vi "add_automatic_steps.vi"(7 "references":T1, 8 "error in (no error)":errorcluster, 11 "automatic_steps":variant) -> (0 "error out":errorcluster)   [LabVIEW 2015, in "repub-dvr_nre.lvlib"]
uses:
  repub-dvr_nre.lvlib
  _controls/references.ctl
  private/_controls/input.ctl
  private/_controls/input_command.ctl
  private/_controls/output.ctl
  private/_controls/data.ctl
  _controls/configuration.ctl
  lv-recipe-machine/private/_controls/recipe_data.ctl
  lv-recipe-machine/public/_controls/mode.ctl
  lv-recipe-machine/public/_controls/manual_state.ctl
  lv-recipe-machine/public/_controls/automatic_state.ctl
  <userlib>/antonio-alexander/lv-waitgroup/public/_controls/api_waitgroup.ctl
  _controls/change.ctl
  lv-recipe-machine/lv-recipe-machine.lvlib
  <userlib>/antonio-alexander/lv-waitgroup/lv-waitgroup.lvlib
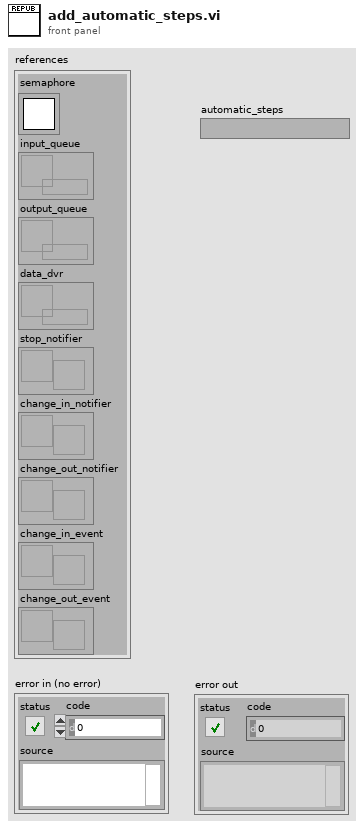
[diagram p1: front panel]
types:
  T1 = typedef "repub-dvr_nre.lvlib/references.ctl" = cluster{"semaphore":T2, "input_queue":refnum<queue>, "output_queue":refnum<queue>, "data_dvr":refnum<data-value>, "stop_notifier":refnum<notifier>, "change_in_notifier":refnum<notifier>, "change_out_notifier":refnum<notifier>, "change_in_event":refnum<user-event>, "change_out_event":refnum<user-event>}
  T2 = typedef "Semaphore RefNum" = refnum<k1>
  T3 = typedef "repub-dvr_nre.lvlib/data.ctl" = cluster{"configuration":T4, "working":cluster{"initialized":bool, "recipe_data":T5, "api_waitgroup":T9}}
  T4 = typedef "repub-dvr_nre.lvlib/configuration.ctl" = cluster{dbl}
  T5 = typedef "lv-recipe-machine.lvlib/recipe_data.ctl" = cluster{"mode":T6, "manual_state":T7, "automatic_state":T8, "step":string, "automatic_recipe":variant, "manual_actions":variant}
  T6 = typedef "lv-recipe-machine.lvlib/mode.ctl" = enum16{"<mode>", "manual", "automatic", "<null>"}
  T7 = typedef "lv-recipe-machine.lvlib/manual_state.ctl" = enum16{"<manual_state>", "failed", "action", "running", "idle", "<null>"}
  T8 = typedef "lv-recipe-machine.lvlib/automatic_state.ctl" = enum16{"<automatic_state>", "failed", "idle", "running", "paused", "transition", "stopped", "<null>"}
  T9 = typedef "lv-waitgroup.lvlib/api_waitgroup.ctl" = cluster{"waitgroups":refnum<data-value>, "waitgroup":string}
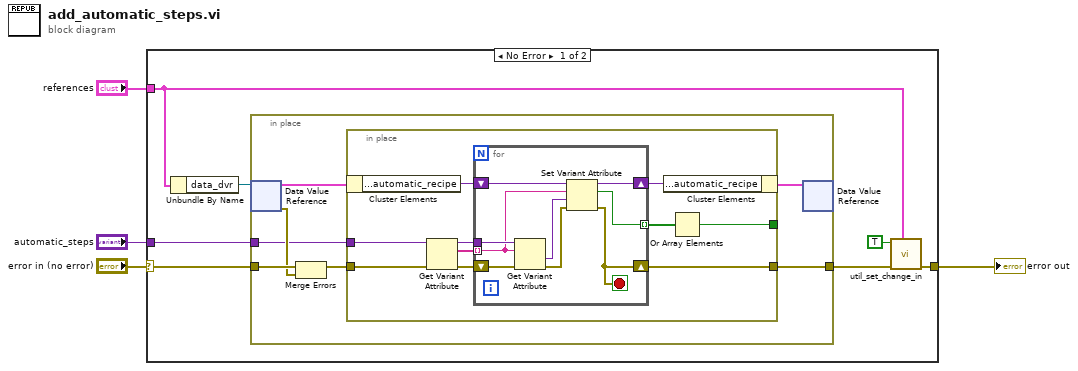
[diagram p0: block diagram]
diagram:
  n1 = case shown="No Error" "error in (no error)" {
    selector: "error in (no error)" -> [w10 w38]
    tunnel: [w8 w38] -> w1
    tunnel: "references" -> [w9 _]
    tunnel: "automatic_steps" -> [w7 _]
    frame No Error {
      n2 = Unbundle By Name(w9) -> ("data_dvr"=w11:refnum<data-value>)
      n3 = in-place {
        in-place-border: [w12] -> w6
        in-place-border: w10 -> [w18]
        in-place-border: w7 -> [w14]
        n4 = in-place-dvr #1(w11) -> (w16:T3, w17:errorcluster)
        n5 = Merge Errors(w18, w17) -> (w13:errorcluster)
        n6 = in-place {
          in-place-border: w14 -> [w26]
          in-place-border: w13 -> [w25]
          in-place-border: [w21] -> w12
          in-place-border: [w19] -> _
          n7 = in-place-cluster #2(w16) -> ("working.recipe_data.automatic_recipe"=w28:variant)
          n8 = Get Variant Attribute(Variant=w26, error in=w25) -> (duplicate Variant=w24:variant, names=w23:string[], error out=w22:errorcluster)  [unwired: 2 in, 1 out]
          n9 = for {
            shift-right: [w36] -> w27
            shift-left: w28 -> [w37]
            tunnel: [w35] -> w20 mode=indexing
            tunnel: w24 -> [w33]
            tunnel: w23 -> [w29] mode=indexing
            shift-right: [w34] -> w21
            shift-left: w22 -> [w32]
            stop <- w34 stop-if-true
            n10 = Get Variant Attribute(Variant=w33, name=w29, error in=w32) -> (value=w30:variant, error out=w31:errorcluster)  [unwired: 1 in, 2 out]
            n11 = Set Variant Attribute(Variant=w37, name=w29, value=w30, error in=w31) -> (Variant out=w36:variant, replaced=w35:bool, error out=w34:errorcluster)
          }
          n12 = in-place-cluster #2("working.recipe_data.automatic_recipe"=w27) -> (w15:T3)
          n13 = Or Array Elements(Boolean array=w20) -> (logical OR=w19:bool)
        }
        n14 = in-place-dvr #1(w15) -> ()  [unwired: 2 out]
      }
      n15 = call "util_set_change_in.vi"("references"=w9, "error in (no error)"=w6, "change"=TRUE) -> ("error out"=w8:errorcluster)  [unwired: 8 in]
    }
    frame Error {
    }
  }
  "error out" <- w1
